vi "Global of computer.vi"() -> ()   [LabVIEW 2012]
panel:
  in  "able to shoot _1":bool
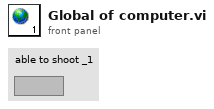
[diagram p1: front panel]
diagram:
